vi "PLL (Hilbert).vi"(0 "input":fxp<+/-,18,1>, 1 "reset":bool, 5 "config":T1={"quiescent frequency"=0.0, "compensation"=0.0, "psd gain"=0, "loop filter"={"order"=1, "cutoff"=4}}, 9 "enable":bool) -> (6 "output":fxp<+/-,48,0>)   [LabVIEW 2017, in "NI PLL IP FPGA.lvlib"]
uses:
  NI PLL IP FPGA.lvlib
  <instrlib>/_niInstr/DSP/v1/Shared/Public/IQ Data.ctl
  <instrlib>/_niInstr/DSP/v1/Shared/niInstr DSP v1 Shared.lvlib
  <instrlib>/_niInstr/DSP/v1/FPGA/Public/Sub VIs/Frequency Shift/Frequency Shift - 1 spc.vi
  <instrlib>/_niInstr/DSP/v1/FPGA/niInstr DSP v1 FPGA.lvlib
  <instrlib>/_niInstr/DSP/v1/Xnodes/Public/Frequency Shift/niInstr DSP v1 Frequency Shift FPGA.xnode
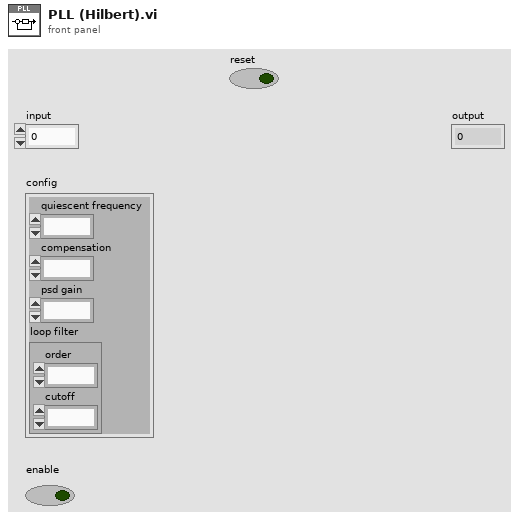
[diagram p1: front panel]
types:
  T1 = cluster{"quiescent frequency":fxp<+/-,48,0>, "compensation":fxp<+/-,18,3>, "psd gain":i16, "loop filter":cluster{"order":i32, "cutoff":i8}}
  T2 = typedef "niInstr DSP v1 Shared.lvlib/IQ Data.ctl" = cluster{"I":fxp<+/-,18,1>, "Q":fxp<+/-,18,1>, "overflow":bool}
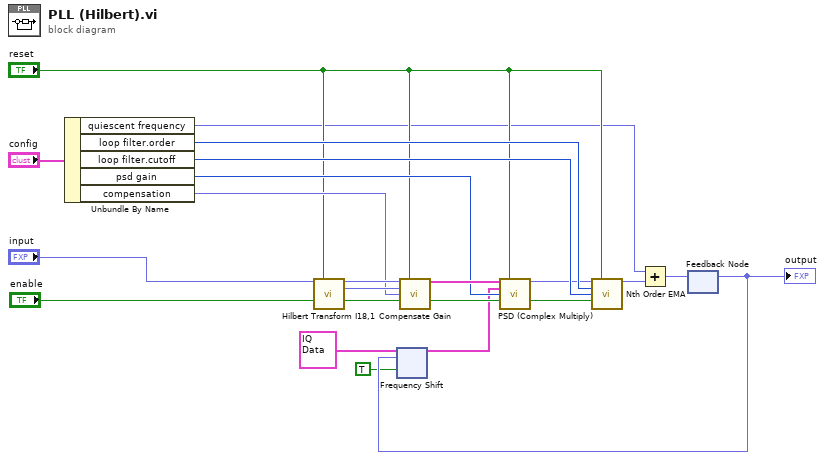
[diagram p0: block diagram]
diagram:
  n1 = Unbundle By Name("config") -> ("quiescent frequency"=w4:fxp<+/-,48,0>, "loop filter.order"=w16:i32, "loop filter.cutoff"=w15:i8, "psd gain"=w12:i16, "compensation"=w11:fxp<+/-,18,3>)
  n2 = call "Hilbert Transform I18,1.vi"("input"="input", "reset"="reset", "input valid"="enable") -> ("i"=w21:fxp<+/-,18,1>, "q"=w20:fxp<+/-,37,3>, "output valid"=w19:bool)  [unwired: 10 in]
  n3 = call "Compensate Gain.vi"("i"=w21, "reset"="reset", "q"=w20, "gain"=w11, "input valid"=w19) -> ("iq data"=w14:T2, "output valid"=w13:bool)  [unwired: 9 in]
  n4 = feedback #1() -> (w3:fxp<+/-,48,0>)  [unwired: 1 in]
  "output" <- w3
  n5 = xnode "Frequency Shift"("data in"=T2 {"I"=0.9999923706054688, "Q"=0.0, "overflow"=FALSE}, "frequency shift"=w3, "input valid"=TRUE) -> ("data out"=w8:T2)  [unwired: 3 in, 2 out]
  n6 = call "PSD (Complex Multiply).vi"("input 0"=w14, "reset"="reset", "input 1"=w8, "k"=w12, "input valid"=w13) -> ("output"=w10:fxp<+/-,48,1>, "output vliad"=w9:bool)  [unwired: 9 in]
  n7 = call "Nth Order EMA.vi"("input"=w10, "reset"="reset", "order"=w16, "n_cutoff"=w15, "input valid"=w9) -> ("output"=w6:fxp<+/-,48,1>)  [unwired: 9 in, 1 out]
  n8 = Add(x=w4, y=w6) -> (x+y=w5:fxp<+/-,48,0>)
  n9 = feedback-in #1(w5) -> ()
